vi "chaincmd Controller.vi"(8 "error in":errorcluster) -> ()   [LabVIEW 2017]
doc: "This VI executes continuously carrying out the current operation and responding to updates or new operations. It will often contain the timing or control code that is difficult to place directly in TeleOp. This VI generally opens all sensors and motors and isolates the rest of the robot code from knowing how the operations are carried out."
uses:
  <vilib>/Rock Robotics/WPI/Framework/Completion Status.ctl
  chaincmd Setpoints.ctl
  chaincmd Operations.ctl
  chaincmd States.ctl
  cube/Implementation/cube Operations.ctl
  tower/Implementation/tower Operations.ctl
  chaincmd Published Globals.vi
  cube/Implementation/cube Published Globals.vi
  tower/Implementation/tower Published Globals.vi
  <vilib>/Rock Robotics/Network Tables/NT Write Boolean.vi
panel:
  out "ChainLastCommandStatus":T1
  out "TestCommandState":T2
  in  "Interactive Values":T3
  out "Current\nCmd":string
  in  "Buttons":cluster{"Execute Cmd":bool, "Abort Cmd":bool}
  out "Command Timing":cluster{"Start Time (ms)":u32, "Iterations":i32}
  out "Status":T1
  # "Tip: It may be helpful to observe inputs and sensor values.\nYou may also want to display tuning or debugging controls."
  # "Interactive Command: You may fill in the settings for a command\nand schedule it with the Execute button. You can observe and abort\nany command while fine tuning the code for the controller."
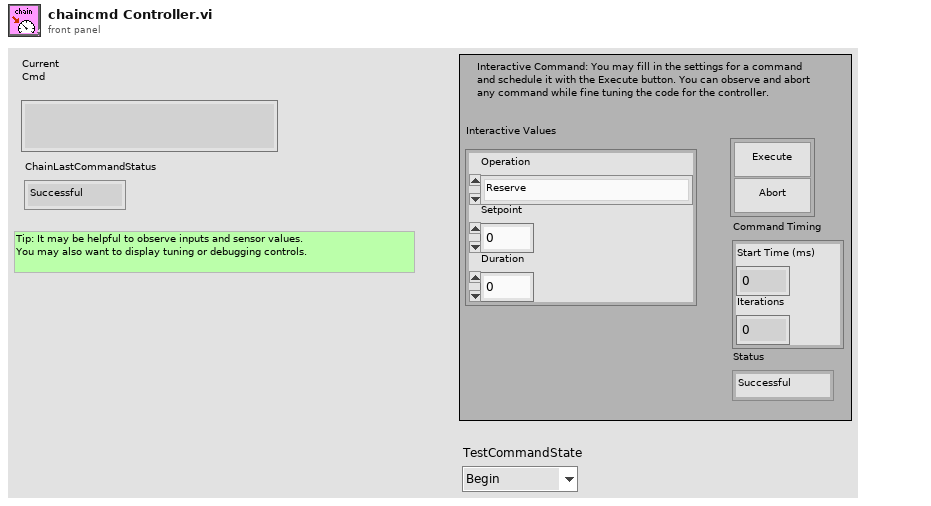
[diagram p1: front panel]
types:
  T1 = typedef "Completion Status.ctl" = enum16{"Successful", "Aborted", "Incomplete"}
  T2 = typedef "chaincmd States.ctl" = enum16{"Begin", "Stage1", "Stage2", "Stage3", "Stage4", "Stage5"}
  T3 = typedef "chaincmd Setpoints.ctl" = cluster{"Operation":T4, "Setpoint":dbl, "Duration":dbl}
  T4 = typedef "chaincmd Operations.ctl" = enum16{"Reserve", "Read Current", "Immediate", "CommandA", "CommandB", "CommandC", "CommandTest"}
  T5 = typedef "Command Status Info.ctl" = cluster{"Name":string, "Status":T1, "notifier out":T6}
  T6 = typedef "Completion Notifier.ctl" = refnum<notifier>
  T7 = cluster{"Current Command":T3, "Command Timing":cluster{"Start Time (ms)":u32, "Iterations":i32}, "Command Arguments":cluster{"Command Info":T5, "Description":string, "Default Command":T3, "queue out":refnum<queue>, "Subsystem Name":string}}
  T8 = typedef "cube Operations.ctl" = enum16{"Reserve", "Read Current", "Immediate", "Chew", "Puke", "Swallow", "Poop", "SpitFast", "SpitSlow"}
  T9 = typedef "tower Operations.ctl" = enum16{"Reserve", "Read Current", "Immediate", "LaunchClimber", "ArmReset", "ArmPosition", "TowerClimbImmediate", "ArmSpitPosition", "ClimbArmMove"}
  T10 = typedef "cube Setpoints.ctl" = cluster{"Operation":T8, "Arm Setpoint":dbl, "Duration":dbl, "Conveyor Setpoint":dbl}
  T11 = typedef "tower Setpoints.ctl" = cluster{"Operation":T9, "Setpoint":dbl, "Duration":dbl}
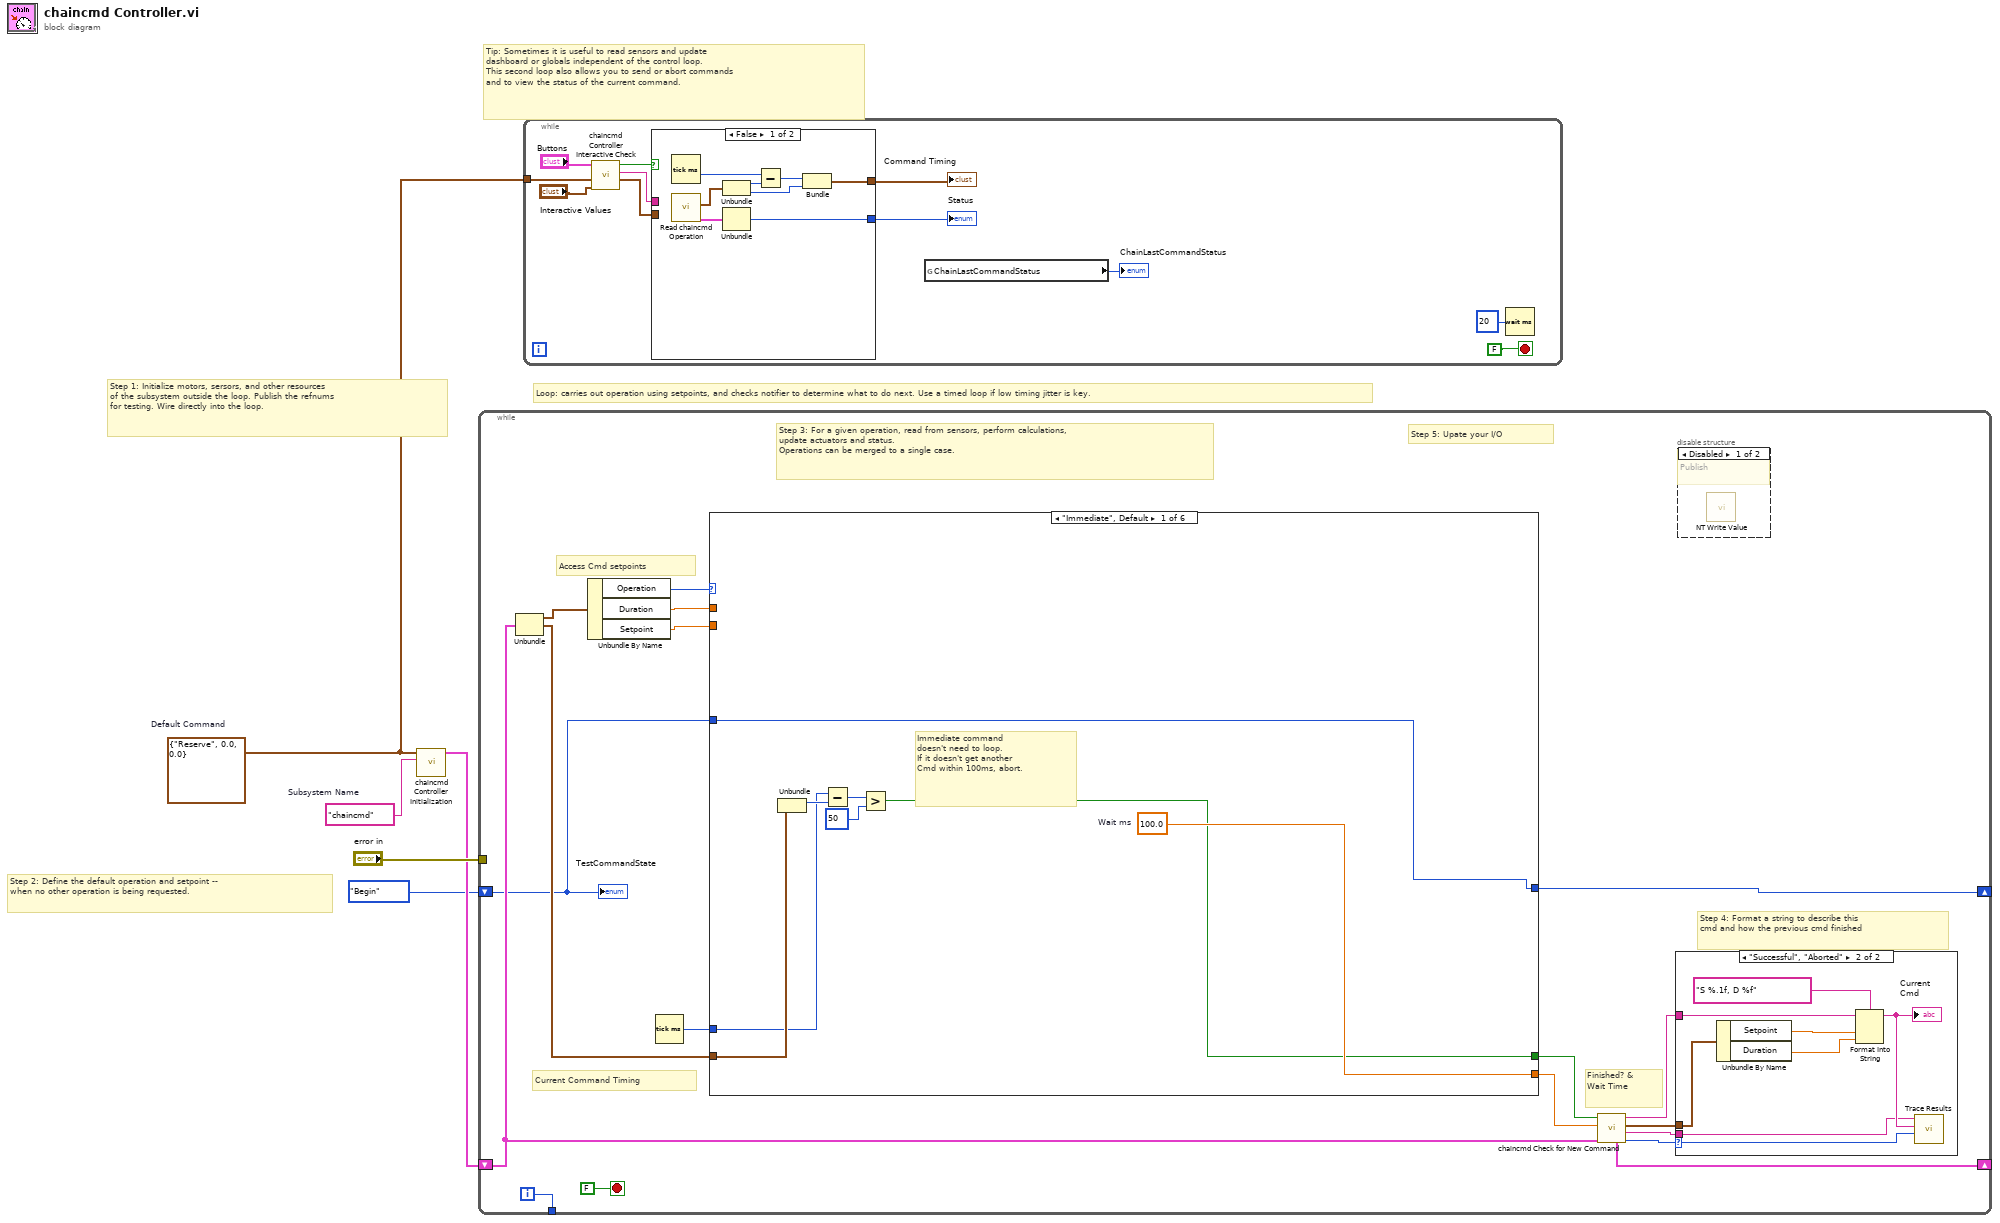
[diagram p0: block diagram]
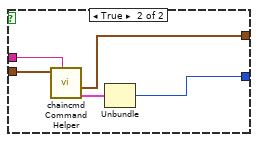
[diagram p2: hidden frame]
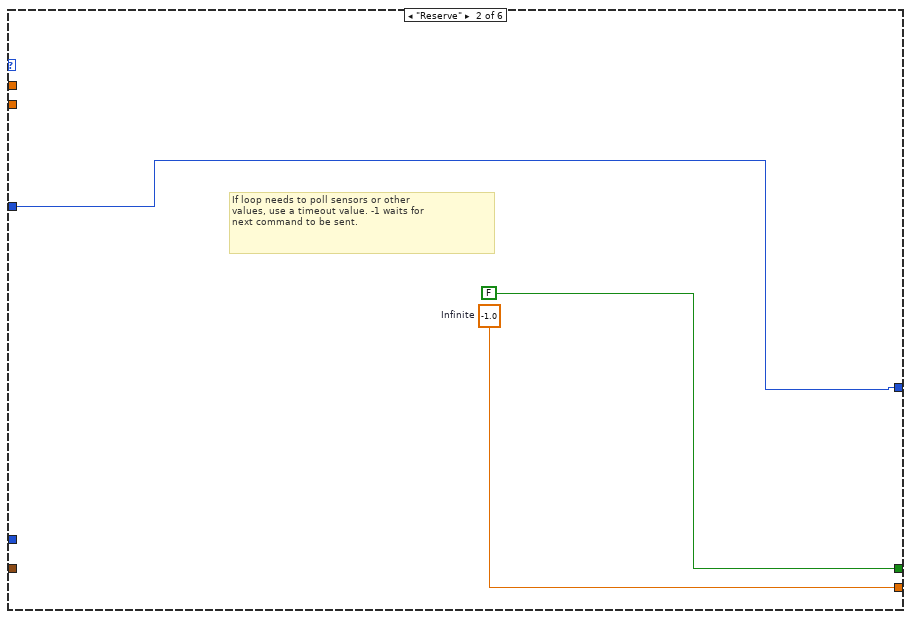
[diagram p5: hidden frame]
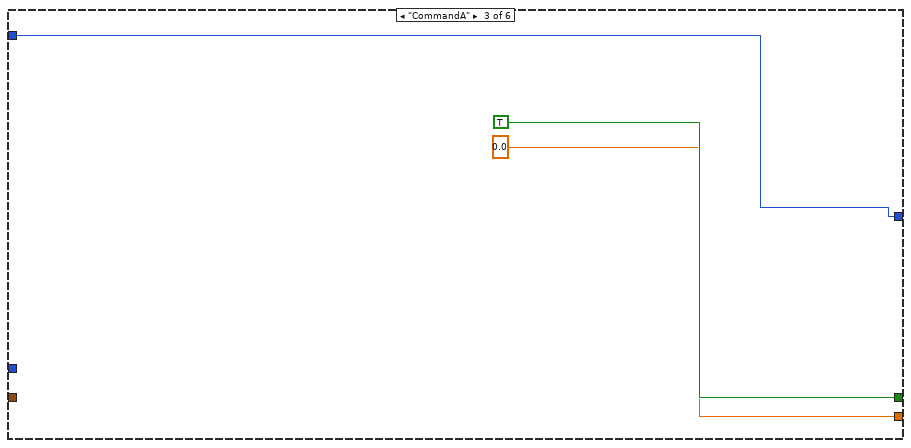
[diagram p6: hidden frame]
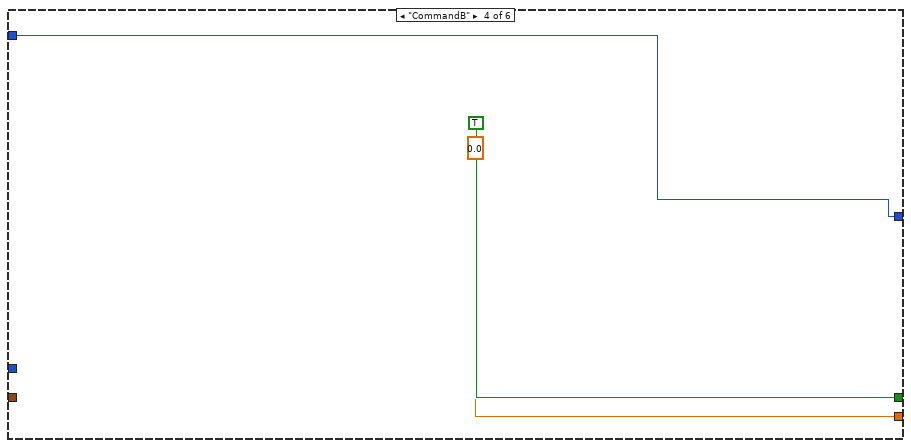
[diagram p7: hidden frame]
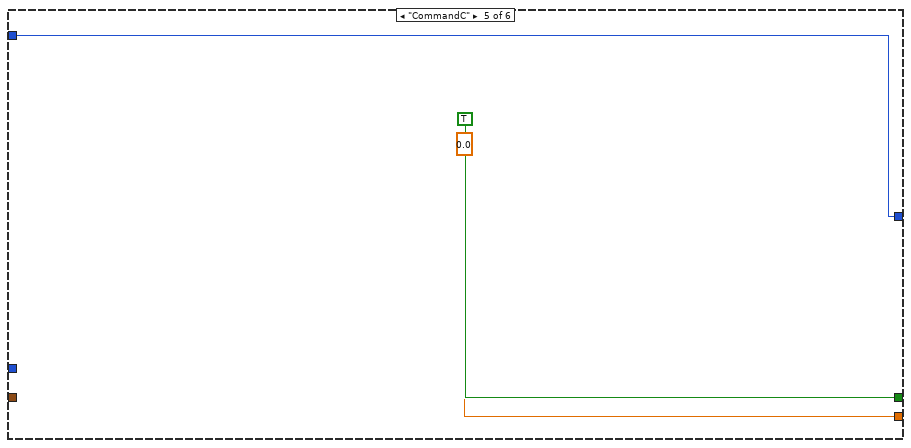
[diagram p8: hidden frame]
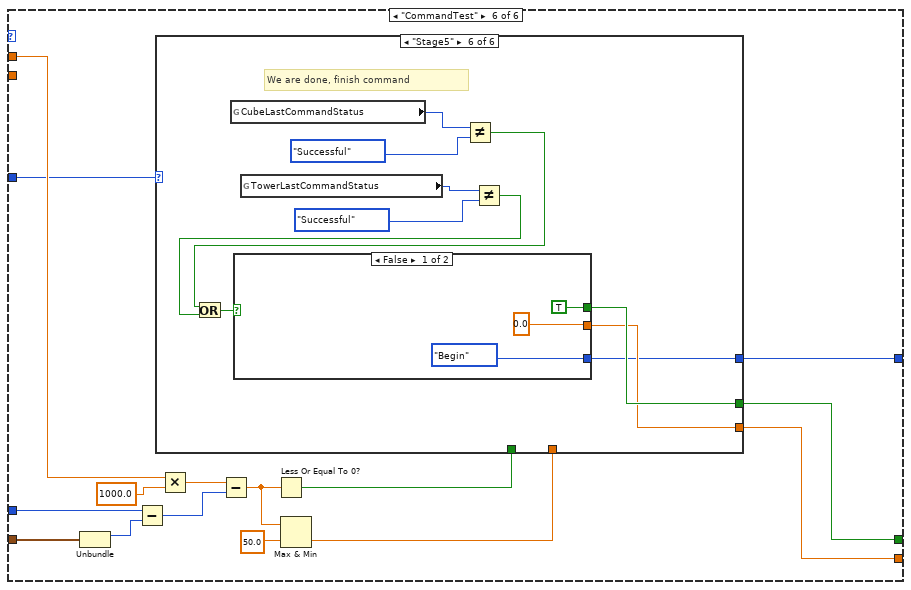
[diagram p9: hidden frame]
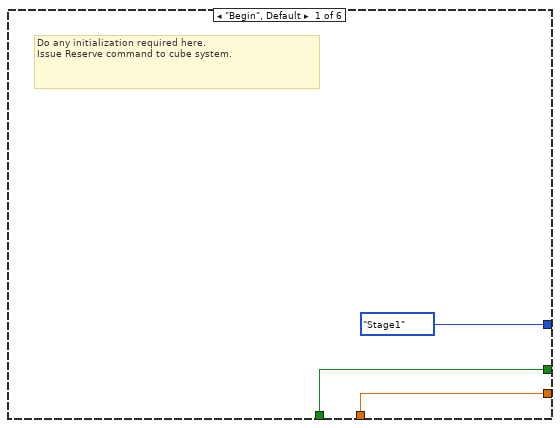
[diagram p10: hidden frame]
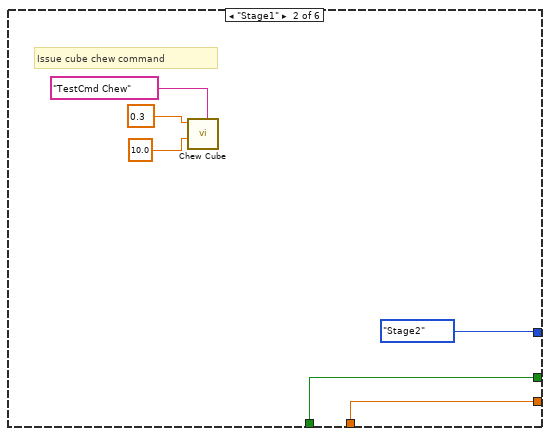
[diagram p11: hidden frame]
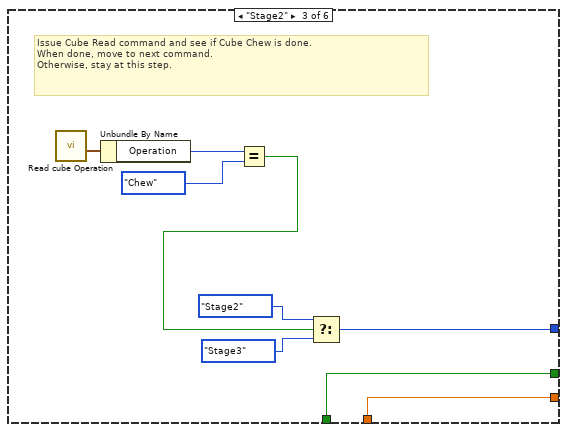
[diagram p12: hidden frame]
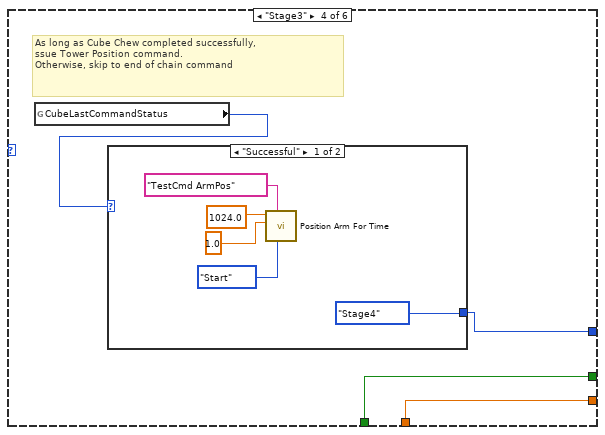
[diagram p13: hidden frame]
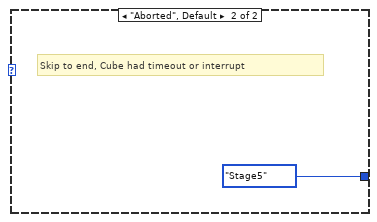
[diagram p14: hidden frame]
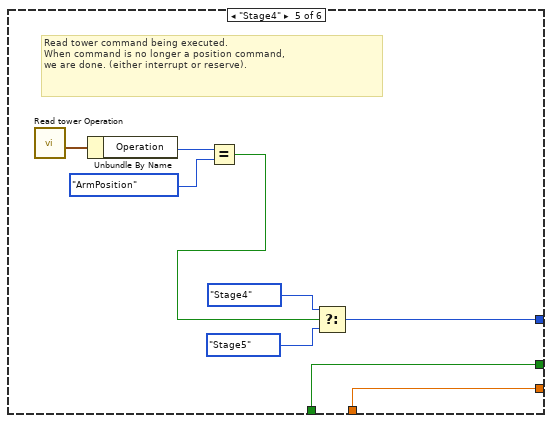
[diagram p15: hidden frame]
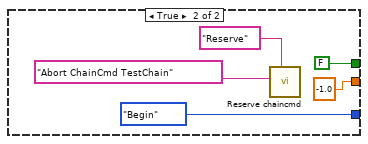
[diagram p16: hidden frame]
diagram:
  w2 = T3 {"Operation"=enum."Reserve", "Setpoint"=0.0, "Duration"=0.0}  # Default Command
  w3 = "chaincmd"  # Subsystem Name
  # "Tip: Sometimes it is useful to read sensors and update\ndashboard or globals independent of the control loop.\nThis second loop also allows you to send or abort commands\nand to view the status of the current command."
  # "Step 2: Define the default operation and setpoint --\nwhen no other operation is being requested."
  # "Step 1: Initialize motors, sersors, and other resources\nof the subsystem outside the loop. Publish the refnums\nfor testing. Wire directly into the loop."
  # "Loop: carries out operation using setpoints, and checks notifier to determine what to do next. Use a timed loop if low timing jitter is key."
  n1 = call "chaincmd Controller Initialization.vi"("Subsystem Name"=w3, "Default Command"=w2) -> ("Current Command"=w4:T7)  [unwired: 9 in]
  n2 = while {
    shift-right: [w15] -> _
    shift-left: w4 -> [w8]
    tunnel: [w22] -> _
    tunnel: "error in" -> [_]
    shift-right: [w7] -> _
    shift-left: chaincmd_States."Begin" ("TestCommandState") -> [w6]
    i -> [w22]
    stop <- FALSE stop-if-true
    # "Step 5: Upate your I/O"
    # "Step 4: Format a string to describe this\ncmd and how the previous cmd finished"
    # "Current Command Timing"
    # "Access Cmd setpoints"
    # "Finished? &\nWait Time"
    # "Step 3: For a given operation, read from sensors, perform calculations,\nupdate actuators and status.\nOperations can be merged to a single case."
    n3 = Unbundle(w8) -> ("Current Command"=w21:T3, "Command Timing"=w17:cluster{"Start Time (ms)":u32, "Iterations":i32})  [unwired: 1 out]
    n4 = Unbundle By Name(w21) -> ("Operation"=w20:T4, "Duration"=w19:dbl, "Setpoint"=w16:dbl)
    n5 = Tick Count (ms)() -> (millisecond timer value=w18:u32)
    n6 = case shown="\"Immediate\", Default" w20 {
      tunnel: [w39 w42 0.0 ("Infinite") 0.0 ("Infinite") 0.0 ("Infinite") w54] -> w13
      tunnel: [w33 FALSE ("ignore previous (F)") TRUE ("ignore previous (F)") TRUE ("ignore previous (F)") TRUE ("ignore previous (F)") w57] -> w14
      tunnel: w17 -> [w35 _ _ _ _ w60]
      tunnel: w19 -> [_ _ _ _ _ w59]
      tunnel: w18 -> [w34 _ _ _ _ w58]
      tunnel: w16 -> [_ _ _ _ _ _]
      tunnel: [w32 w40 w43 w46 w49 w53] -> w7
      tunnel: w6 -> [w32 w40 w43 w46 w49 w52]
      frame "Immediate", Default {
        w39 = 100.0  # Wait ms
        # "Immediate command\ndoesn't need to loop.\nIf it doesn't get another\nCmd within 100ms, abort."
        n7 = Unbundle(w35) -> ("Start Time (ms)"=w38:u32)  [unwired: 1 out]
        n8 = Subtract(x=w34, y=w38) -> (x-y=w37:u32)
        n9 = Greater?(x=w37, y=u8 50 ("Left Motor")) -> (0:w33:bool)
      }
      frame "Reserve" {
        w42 = -1.0  # Infinite
        # "If loop needs to poll sensors or other\nvalues, use a timeout value. -1 waits for\nnext command to be sent."
      }
      frame "CommandA" {
      }
      frame "CommandB" {
      }
      frame "CommandC" {
      }
      frame "CommandTest" {
        n10 = Unbundle(w60) -> ("Start Time (ms)"=w63:u32)  [unwired: 1 out]
        n11 = Subtract(x=w58, y=w63) -> (x-y=w66:u32)
        n12 = Multiply(x=w59, y=1000.0) -> (x*y=w65:dbl)
        n13 = Subtract(x=w65, y=w66) -> (x-y=w62:dbl)
        n14 = Less Or Equal To 0?(x=w62) -> (x <= 0?=w56:bool)
        n15 = Max & Min(x=w62, y=50.0) -> (min(x,y)=w55:dbl)  [unwired: 1 out]
        n16 = case shown="\"Stage5\"" w52 {
          tunnel: [chaincmd_States."Stage1" ("TestCommandState") chaincmd_States."Stage2" ("TestCommandState") w78 w87 w98 w104] -> w53
          tunnel: [w69 w73 w76 w85 w96 w110] -> w57
          tunnel: [w68 w74 w77 w86 w97 w109] -> w54
          tunnel: w56 -> [w69 w73 w76 w85 w96 _]
          tunnel: w55 -> [w68 w74 w77 w86 w97 _]
          frame "Begin", Default {
            # "Do any initialization required here.\nIssue Reserve command to cube system."
          }
          frame "Stage1" {
            # "Issue cube chew command"
            n17 = call "Chew Cube.vi"("Arm Setpoint"=0.3 ("Setpoint"), "Duration (s)"=10.0, "Description"="TestCmd Chew") -> ()  [unwired: 7 in, 1 out]
          }
          frame "Stage2" {
            # "Issue Cube Read command and see if Cube Chew is done.\nWhen done, move to next command.\nOtherwise, stay at this step."
            n18 = call "Read cube Operation.vi"() -> ("SubSystem Data"=w84:T10)  [unwired: 9 in, 2 out]
            n19 = Unbundle By Name(w84) -> ("Operation"=w83:T8)
            n20 = Equal?(x=w83, y=cube_Operations."Chew") -> (x = y?=w81:bool)
            n21 = Select(t=chaincmd_States."Stage2" ("TestCommandState"), s=w81, f=chaincmd_States."Stage3" ("TestCommandState")) -> (s? t:f=w78:T2)
          }
          frame "Stage3" {
            # "As long as Cube Chew completed successfully,\nssue Tower Position command. \nOtherwise, skip to end of chain command"
            n22 = global read "cube Published Globals.vi" "CubeLastCommandStatus"() -> (w88:T1)
            n23 = case shown="\"Successful\"" w88 {
              tunnel: [chaincmd_States."Stage4" ("TestCommandState") chaincmd_States."Stage5" ("TestCommandState")] -> w87
              frame "Successful" {
                n24 = call "Position Arm For Time.vi"("Synchronization"=enum16{"Start", "Wait"}."Start", "Description"="TestCmd ArmPos", "Duration (s)"=1.0, "Setpoint"=1024.0) -> ()  [unwired: 7 in, 1 out]
              }
              frame "Aborted", Default {
                # "Skip to end, Cube had timeout or interrupt"
              }
            }
          }
          frame "Stage4" {
            # "Read tower command being executed.\nWhen command is no longer a position command,\nwe are done. (either interrupt or reserve)."
            n25 = call "Read tower Operation.vi"() -> ("SubSystem Data"=w103:T11)  [unwired: 9 in, 2 out]
            n26 = Unbundle By Name(w103) -> ("Operation"=w102:T9)
            n27 = Equal?(x=w102, y=tower_Operations."ArmPosition" ("Operation")) -> (x = y?=w101:bool)
            n28 = Select(t=chaincmd_States."Stage4" ("TestCommandState"), s=w101, f=chaincmd_States."Stage5" ("TestCommandState")) -> (s? t:f=w98:T2)
          }
          frame "Stage5" {
            # "We are done, finish command"
            n29 = global read "cube Published Globals.vi" "CubeLastCommandStatus"() -> (w107:T1)
            n30 = global read "tower Published Globals.vi" "TowerLastCommandStatus"() -> (w105:T1)
            n31 = Not Equal?(x=w107, y=enum16{"Successful", "Aborted", "Incomplete"}."Successful" ("CubeLastCommandStatus")) -> (x != y?=w112:bool)
            n32 = Not Equal?(x=w105, y=enum16{"Successful", "Aborted", "Incomplete"}."Successful" ("TowerLastCommandStatus")) -> (x != y?=w111:bool)
            n33 = Or(x=w112, y=w111) -> (x .or. y?=w113:bool)
            n34 = case shown="False" w113 {
              tunnel: [chaincmd_States."Begin" ("TestCommandState") chaincmd_States."Begin" ("TestCommandState")] -> w104
              tunnel: [TRUE FALSE] -> w110
              tunnel: [0.0 -1.0] -> w109
              frame False {
              }
              frame True {
                n35 = call "Reserve chaincmd.vi"("Description"="Reserve", "Command Name"="Abort ChainCmd TestChain") -> ()  [unwired: 9 in, 1 out]
              }
            }
          }
        }
      }
    }
    n36 = call "chaincmd Check for New Command.vi"("Current Command"=w8, "Wait time (ms)"=w13, "Finished?"=w14) -> ("Completion"=w9:T1, "Subsystem Name"=w10:string, "Current Command"=w11:T3, "Initial Trace String"=w12:string, "NextCommand"=w15:T7)  [unwired: 4 in]
    n37 = case shown="\"Successful\", \"Aborted\"" w9 {
      selector: w9 -> [_ w31]
      tunnel: w12 -> [_ w27]
      tunnel: w11 -> [_ w28]
      tunnel: w10 -> [_ w24]
      frame "Incomplete", Default {
        # "Continuing current command"
      }
      frame "Successful", "Aborted" {
        # "Report and setup for next command"
        n38 = Unbundle By Name(w28) -> ("Setpoint"=w30:dbl, "Duration"=w25:dbl)
        n39 = Format Into String(format string="S %.1f, D %f", initial string=w27, w30, w25) -> (resulting string=w26:string)  [unwired: 1 in, 1 out]
        "Current\nCmd" <- w26
        n40 = call <vilib>:"Trace Results.vi"("Status of previous command"=w31, "Description"=w26, "Subsystem"=w24) -> ()  [unwired: 9 in]
      }
    }
    n41 = disable-structure shown="Disabled" {
      frame Disabled {
        # "Publish"
        n42 = call-poly <vilib>:"NT Write Value.vi"() -> ()  [unwired: 11 in, 1 out]
      }
      frame Enabled {
      }
    }
    "TestCommandState" <- w6
  }
  n43 = while {
    tunnel: w2 -> [w129]
    stop <- FALSE stop-if-true
    n44 = call "chaincmd Controller Interactive Check.vi"("Interactive Command in"="Interactive Values", "Default Command"=w129, "Buttons"="Buttons") -> ("Interactive Command out"=w126:T3, "Trace String"=w127:string, "Schedule"=w128:bool)  [unwired: 6 in]
    n45 = case shown="False" w128 {
      tunnel: [w140 w145] -> w125
      tunnel: w126 -> [_ w143]
      tunnel: [w136 w141] -> w124
      tunnel: w127 -> [_ w144]
      frame False {
        n46 = Tick Count (ms)() -> (millisecond timer value=w135:u32)
        n47 = call "Read chaincmd Operation.vi"() -> ("Command Info"=w134:T5, "Command Timing"=w133:cluster{"Start Time (ms)":u32, "Iterations":i32})  [unwired: 9 in, 1 out]
        n48 = Unbundle(w133) -> ("Start Time (ms)"=w139:u32, "Iterations"=w137:i32)
        n49 = Unbundle(w134) -> ("Status"=w140:T1)  [unwired: 2 out]
        n50 = Subtract(x=w135, y=w139) -> (x-y=w138:u32)
        n51 = Bundle(w138, "Iterations"=w137) -> (w136:cluster{u32, "Iterations":i32})  [unwired: 1 in]
      }
      frame True {
        n52 = call "chaincmd Command Helper.vi"("Description"=w144, "SubSystem Data"=w143) -> ("Command Info Out"=w142:T5, "Command Timing"=w141:cluster{"Start Time (ms)":u32, "Iterations":i32})  [unwired: 7 in, 1 out]
        n53 = Unbundle(w142) -> ("Status"=w145:T1)  [unwired: 2 out]
      }
    }
    "Status" <- w125
    "Command Timing" <- w124
    n54 = global read "chaincmd Published Globals.vi" "ChainLastCommandStatus"() -> (→"ChainLastCommandStatus":T1)
    n55 = Wait (ms)(milliseconds to wait=u32 20) -> ()  [unwired: 1 out]
  }
